vi "Expiring Cache.vi"(7 "Directive (Not Specified)":T1, 8 "error in (no error)":errorcluster, 10 "Expires":timestamp, 11 "Response in":refnum<class "Response.lvclass">) -> (0 "error out":errorcluster, 3 "Response out":refnum<class "Response.lvclass">)   [LabVIEW 2020, in "HTTP Utils.lvlib" / "Response.lvclass"]
uses:
  Response.lvclass
  Cache Directive.ctl
  HTTP Utils.lvlib
  Cache Params.ctl
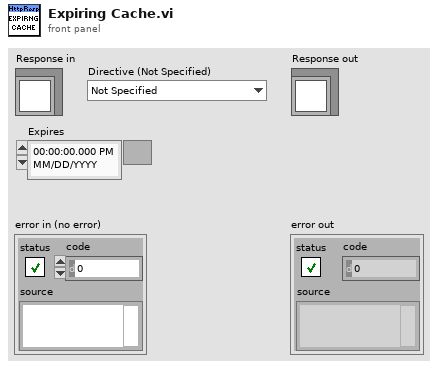
[diagram p1: front panel]
types:
  T1 = typedef "HTTP Utils.lvlib/Cache Directive.ctl" = enum16{"Not Specified", "None (no-store)", "Always Validate (no-cache)", "Private Only (private)", "Always Allow (public)"}
  T2 = typedef "HTTP Utils.lvlib/Cache Params.ctl" = cluster{"Enabled":bool, "Directive":T1, "Max Age":i32, "Immutable":bool, "Last Modified":timestamp, "Expires":timestamp, "ETag":string, "Weak ETag":bool}
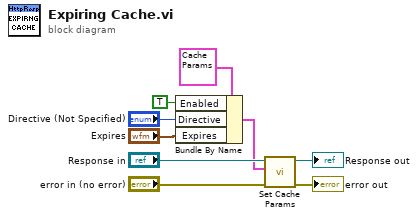
[diagram p0: block diagram]
diagram:
  n1 = Bundle By Name(cluster=T2 {"Enabled"=FALSE, "Directive"=enum."None (no-store)", "Max Age"=0, "Immutable"=FALSE, "Last Modified"=timestamp(0 s since 1904-01-01), "Expires"=timestamp(0 s since 1904-01-01), "ETag"="", "Weak ETag"=FALSE} ("Cache Params"), "Enabled"=TRUE, "Directive"="Directive (Not Specified)", "Expires"="Expires") -> (w4:T2)
  n2 = call "Set Cache Params.vi"("error in (no error)"="error in (no error)", "Cache Params"=w4, "Response in"="Response in") -> ("error out"=→"error out":errorcluster, "Response out"=→"Response out":refnum<class "Response.lvclass">)  [unwired: 7 in]
